vi "Test Empty Folders.vi"(4 "Folders to Exclude":string[](array[string]), 8 "error in (no error)":errorcluster, 11 "Folder Path":path=path "C:/temp/TDMS rename") -> (0 "error out":errorcluster, 2 "ContainsEmptyFolder(s)?":bool)   [LabVIEW 2020]
doc: "This VI will delete all empty folders, under a given folder path.\n\n-------------\nPackage Information\n\nProduct Name: Hooovahh File IO\nPackage File Name: Hooovahh_File_IO\nPackage Version: 1.0.2.4\nMinimum LabVIEW Version: 20.0"
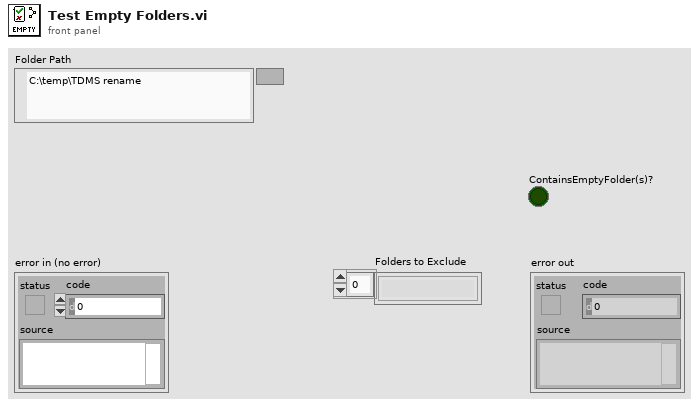
[diagram p1: front panel]
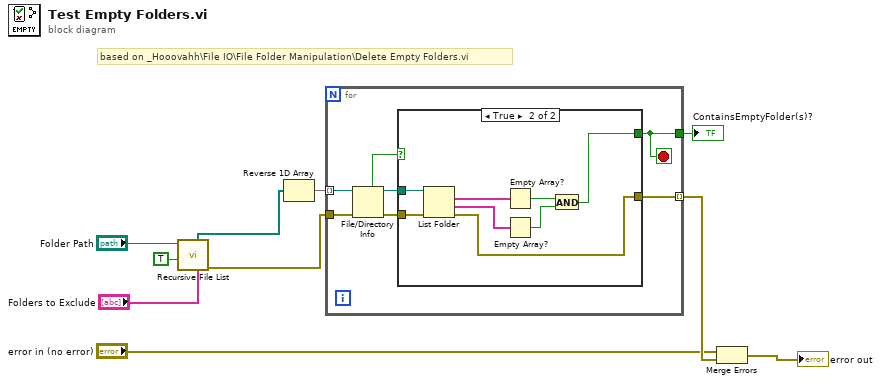
[diagram p0: block diagram]
diagram:
  # "based on _Hooovahh\\File IO\\File Folder Manipulation\\Delete Empty Folders.vi"
  n1 = call <vilib>:"Recursive File List.vi"("Folders to Exclude"="Folders to Exclude", "Continue Recursing on Error? (F)"=TRUE, "Folder Path"="Folder Path") -> ("error out"=w3:errorcluster, "All Folders"=w4:path[])  [unwired: 4 in, 3 out]
  n2 = Reverse 1D Array(array=w4) -> (reversed array=w9:path[])
  n3 = for {
    tunnel: w9 -> [w17] mode=indexing
    tunnel: w3 -> [w14]
    tunnel: [w12] -> w8 mode=indexing
    tunnel: [w11] -> w6
    stop <- w11 stop-if-true
    n4 = File/Directory Info(path=w17, error in=w14) -> (path out=w16:path, directory=w15:bool, error out=w13:errorcluster)  [unwired: 4 out]
    n5 = case shown="True" w15 {
      tunnel: w16 -> [_ w26]
      tunnel: w13 -> [w18 w21]
      tunnel: [w18 w19] -> w12
      tunnel: [_ w20] -> w11
      frame False {
      }
      frame True {
        n6 = List Folder(path=w26, error in=w21) -> (filenames=w25:string[], folder names=w23:string[], error out=w19:errorcluster)  [unwired: 2 in, 1 out]
        n7 = Empty Array?(array=w25) -> (empty?=w24:bool)
        n8 = Empty Array?(array=w23) -> (empty?=w22:bool)
        n9 = And(x=w24, y=w22) -> (x .and. y?=w20:bool)
      }
    }
  }
  "ContainsEmptyFolder(s)?" <- w6
  n10 = Merge Errors("error in (no error)", w8) -> (→"error out":errorcluster)
